vi "IsDAQmxinstalled.vi"(8 "Error In":errorcluster) -> (0 "Error Out":errorcluster, 3 "Is DAQmx Installed":bool)   [LabVIEW 2014]
uses:
  <vilib>/Utility/sysdir.llb/System Directory Type.ctl
panel:
  out "?":string
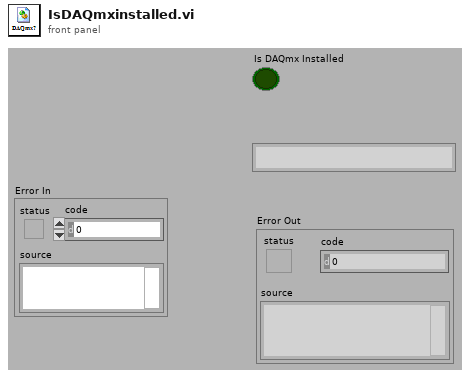
[diagram p1: front panel]
types:
  T1 = typedef "System Directory Type.ctl" = i32
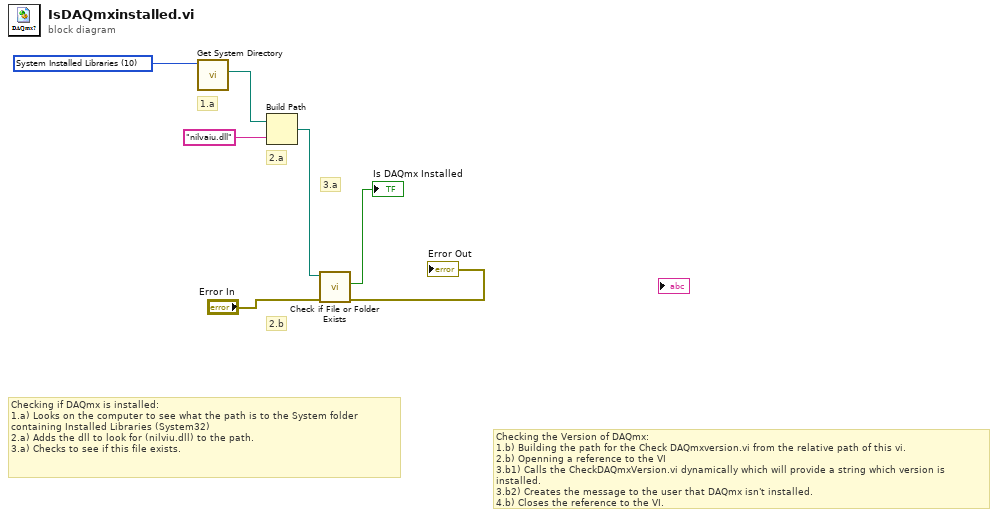
[diagram p0: block diagram]
diagram:
  w7 = T1 10 items=["User Home", "User Desktop", "User Documents", "User Application Data", "User Preferences", "User Temporary", "Public Documents", "Public Application Data", "Public Preferences", "System Core Libraries", "System Installed Libraries", "Application Files", "Boot Volume Root"] ("system directory type")
  # "Checking the Version of DAQmx:\n1.b) Building the path for the Check DAQmxversion.vi from the relative path of this vi.\n2.b) Openning a reference to the VI\n3.b1) Calls the CheckDAQmxVersion.vi dynamically which will provide a string which version is installed.\n3.b2) Creates the message to the user that DAQmx isn't installed.\n4.b) Closes the reference to the VI."
  # "2.b"
  # "Checking if DAQmx is installed:\n1.a) Looks on the computer to see what the path is to the System folder containing Installed Libraries (System32)\n2.a) Adds the dll to look for (nilviu.dll) to the path.\n3.a) Checks to see if this file exists."
  # "3.a"
  # "2.a"
  # "1.a"
  n1 = call <vilib>:"Get System Directory.vi"("system directory type"=w7) -> ("system directory"=w6:path)  [unwired: 10 in]
  n2 = Build Path(base path=w6, name or relative path="nilvaiu.dll") -> (appended path=w4:path)
  n3 = call <vilib>:"Check if File or Folder Exists.vi"("error in (no error)"="Error In", "path"=w4) -> ("error out"=→"Error Out":errorcluster, "file or folder exists?"=→"Is DAQmx Installed":bool)  [unwired: 7 in, 1 out]
